vi "Fetch Waveform.vi"(8 "error in":errorcluster, 10 "Channel":i32, 11 "Rigol DS1054 in":refnum<class "Rigol DS1054.lvclass">) -> (0 "error out":errorcluster, 3 "Rigol DS1054 out":refnum<class "Rigol DS1054.lvclass">)   [LabVIEW 2023, in "RIGOL DS1054.lvlib" / "Rigol DS1054.lvclass"]
uses:
  Rigol DS1054.lvclass
  Rigol DS1054.lvclass/Rigol DS1054.ctl
  <instrlib>/RIGOL DS1000 Series/RIGOL DS1000 Series.lvlib
  Scope Base/Scope Base.lvclass
  D:/git/HAL/Scope VISA/Scope VISA.lvclass
  D:/git/HAL/Scope Base/Scope Base.lvclass
  D:/git/HAL/Hardware_class/Instrument.lvclass
  D:/git/HAL/Interfaces/IScope/IScope.lvclass
  D:/git/HAL/Devices/Rigol DS1054/Rigol DS1054.lvclass
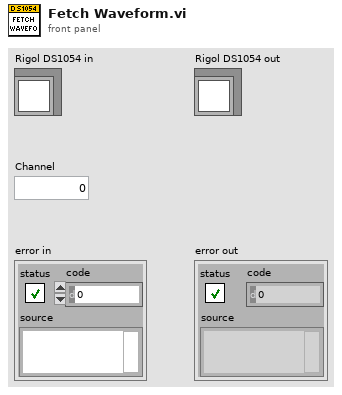
[diagram p1: front panel]
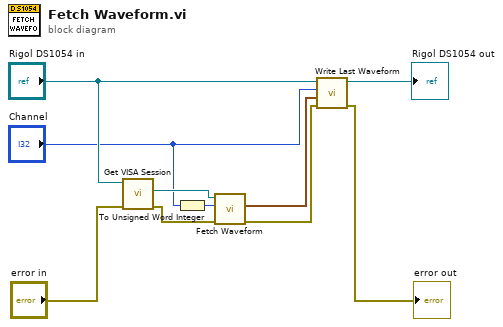
[diagram p0: block diagram]
diagram:
  n1 = call-dynamic "Get VISA Session.vi"("error in"="error in", "Scope VISA in"="Rigol DS1054 in") -> ("error out"=w9:errorcluster, "VISA session"=w8:refnum<visa-resource-name>)  [unwired: 7 in, 1 out]
  n2 = To Unsigned Word Integer(number="Channel") -> (unsigned 16bit integer=w7:u16)
  n3 = call <instrlib>:"Fetch Waveform.vi"("error in (no error)"=w9, "Channel (0: Channel 1)"=w7, "VISA resource name"=w8) -> ("error out"=w3:errorcluster, "Waveform Data"=w4:waveform(dbl))  [unwired: 6 in, 1 out]
  n4 = call "Write Last Waveform.vi"("error in (no error)"=w3, "Last Waveform"=w4, "Channel"="Channel", "Scope Base in"="Rigol DS1054 in") -> ("error out"=→"error out":errorcluster, "Scope Base out"=→"Rigol DS1054 out":refnum<class "Rigol DS1054.lvclass">)  [unwired: 6 in]
